vi "DefaultConstructor.vi"(0 "reference in":refnum<class "G#MethodTemplates.lvclass">, 5 "error in (no error)":errorcluster) -> (14 "reference out":refnum<class "G#MethodTemplates.lvclass">, 19 "error out":errorcluster)   [LabVIEW 2017, in "G#MethodTemplates.lvclass"]
uses:
  <vilib>/addons/_AddQ/G#Templates/G#MethodTemplates/G#MethodTemplates.lvclass
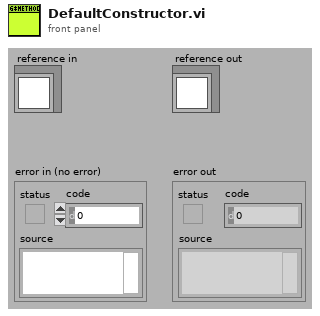
[diagram p1: front panel]
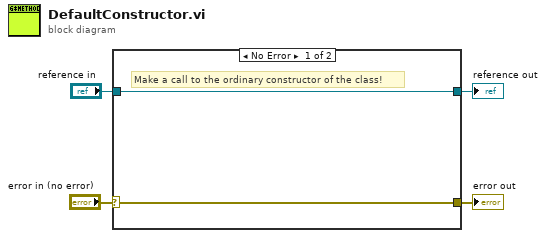
[diagram p0: block diagram]
diagram:
  n1 = case shown="No Error" "error in (no error)" {
    selector: "error in (no error)" -> [w5 w8]
    tunnel: [w5 w8] -> w3
    tunnel: [w6 w7] -> w1
    tunnel: "reference in" -> [w6 w7]
    frame No Error {
      # "Make a call to the ordinary constructor of the class!"
    }
    frame Error {
    }
  }
  "error out" <- w3
  "reference out" <- w1
